vi "Set Points to XML.vi"() -> (0 "XML Data":string)   [LabVIEW 2013]
uses:
  Types/Set Points.ctl
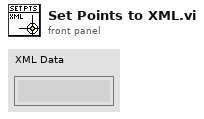
[diagram p1: front panel]
types:
  T1 = typedef "Set Points.ctl" = cluster{"X Position Set-point":dbl, "Y Position Set-point":dbl, "Z Position Set-point":dbl, "Z Scan Set-point":dbl, "Version":string}
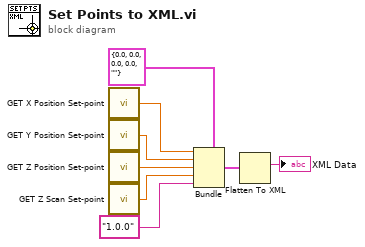
[diagram p0: block diagram]
diagram:
  n1 = call "GET X Position Set-point.vi"() -> ("X Position Set-point"=w5:dbl)
  n2 = call "GET Y Position Set-point.vi"() -> ("Y Position Set-point"=w3:dbl)
  n3 = call "GET Z Position Set-point.vi"() -> ("Z Position Set-point"=w4:dbl)
  n4 = call "GET Z Scan Set-point.vi"() -> ("Z Scan Set-point"=w6:dbl)
  n5 = Bundle(cluster=T1 {"X Position Set-point"=0.0, "Y Position Set-point"=0.0, "Z Position Set-point"=0.0, "Z Scan Set-point"=0.0, "Version"=""} ("Set Points"), "X Position Set-point"=w5, "Y Position Set-point"=w3, "Z Position Set-point"=w4, "Z Scan Set-point"=w6, "Version"="1.0.0") -> (w8:T1)
  n6 = Flatten To XML(anything=w8) -> (xml string=→"XML Data":string)
